vi "PH_PP_CurrentMeas_RT_Startup.vi"() -> ()   [LabVIEW 2014]
uses:
  <vilib>/Utility/error.llb/DialogType.ctl
  <vilib>/DAQmx/create/channels.llb/DAQmx Create Channel (AI-Voltage-Basic).vi
  <vilib>/DAQmx/configure/timing.llb/DAQmx Timing (Sample Clock).vi
  <vilib>/DAQmx/configure/trigger.llb/DAQmx Start Trigger (Analog Edge).vi
  <vilib>/DAQmx/read.llb/DAQmx Read (Analog 1D Wfm NChan NSamp).vi
panel:
  out "Error Port 6343":string
  out "Status Port 6343":string
  out "Error Port 6342":string
  out "Status Port 6342":string
  in  "NI6071E Command Cluster":T1
  in  "error in":errorcluster
  out "Status Port 6341":string
  out "Error Port 6341":string
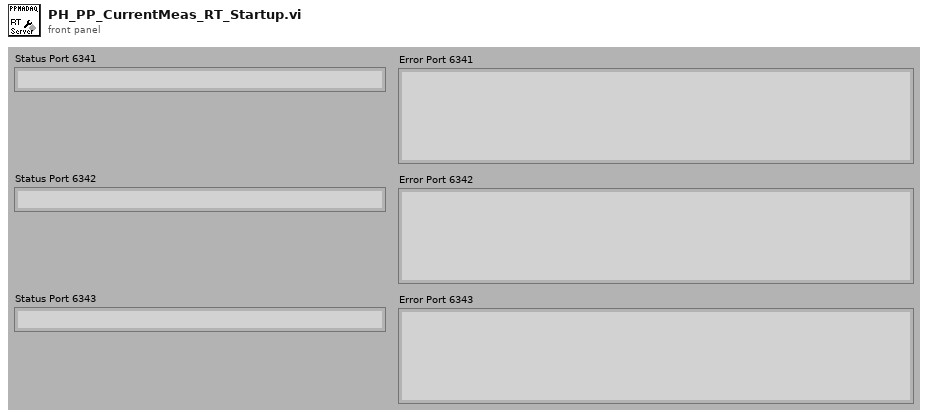
[diagram p1: front panel]
types:
  T1 = cluster{"Command":string, "Data":string, "error out":errorcluster}
  T2 = typedef "DialogType.ctl" = u16
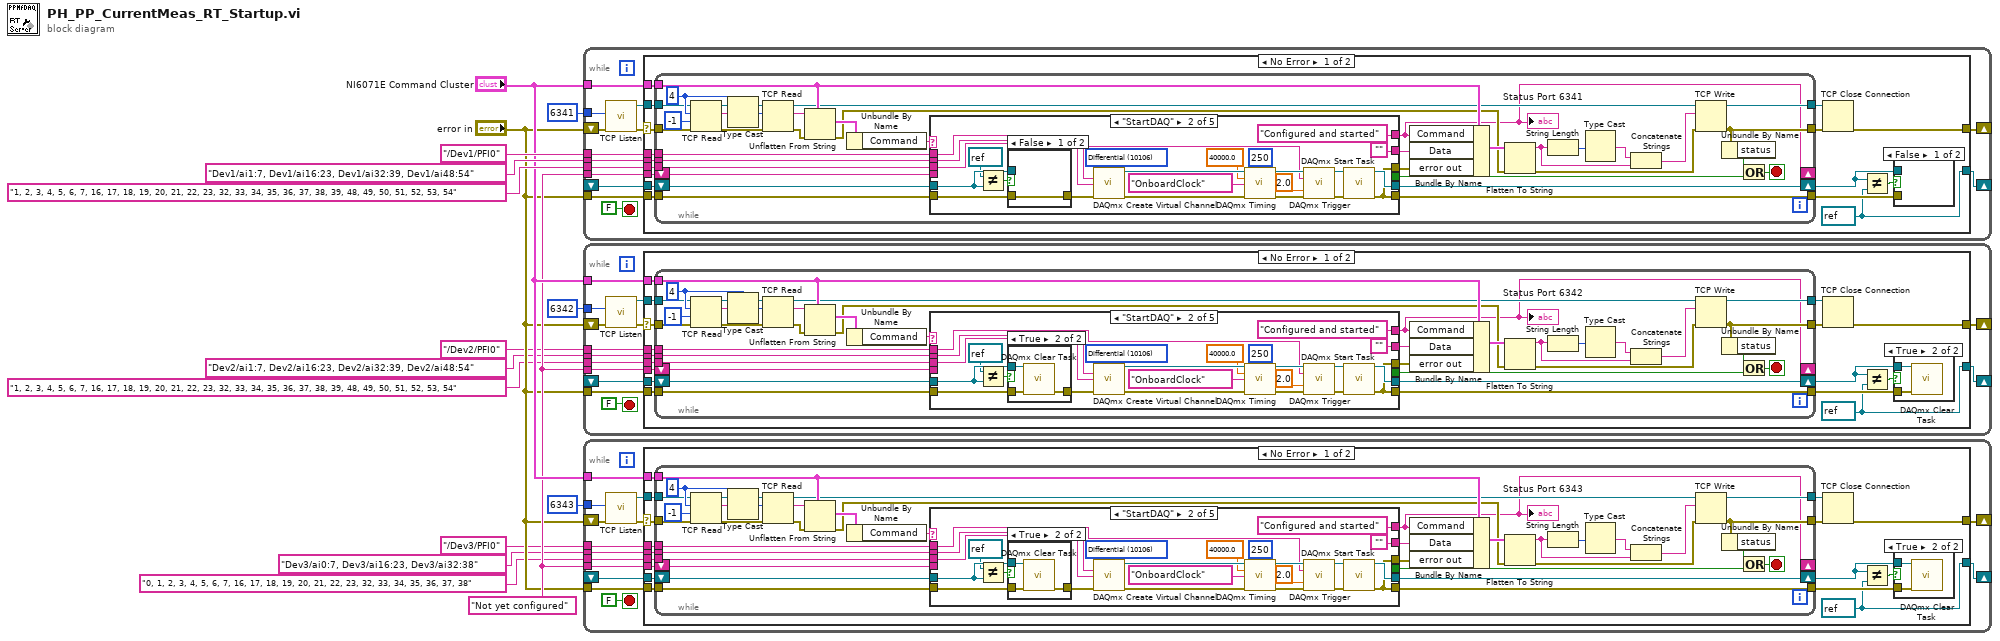
[diagram p0: block diagram]
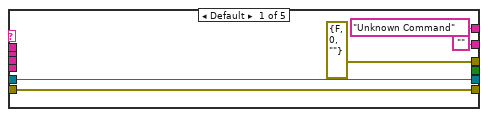
[diagram p3: hidden frame]
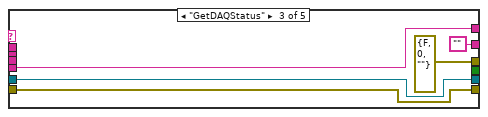
[diagram p5: hidden frame]
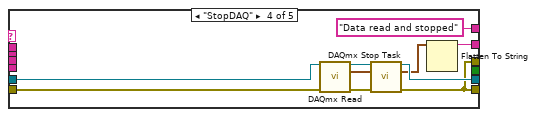
[diagram p6: hidden frame]
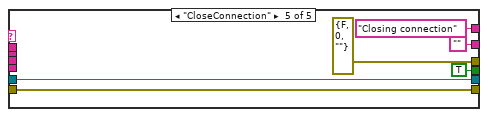
[diagram p7: hidden frame]
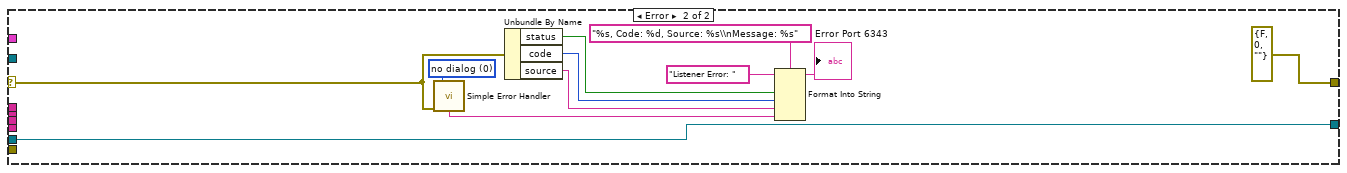
[diagram p8: hidden frame]
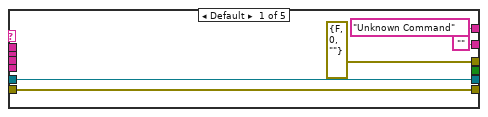
[diagram p10: hidden frame]
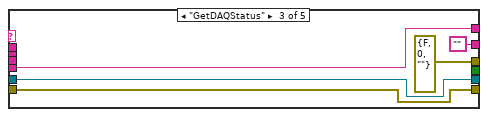
[diagram p12: hidden frame]
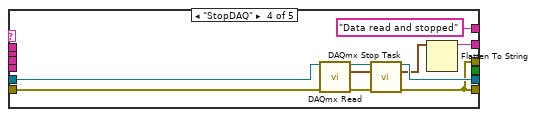
[diagram p13: hidden frame]
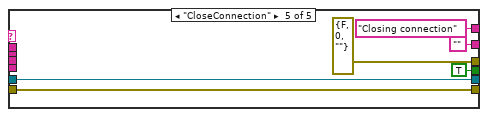
[diagram p14: hidden frame]
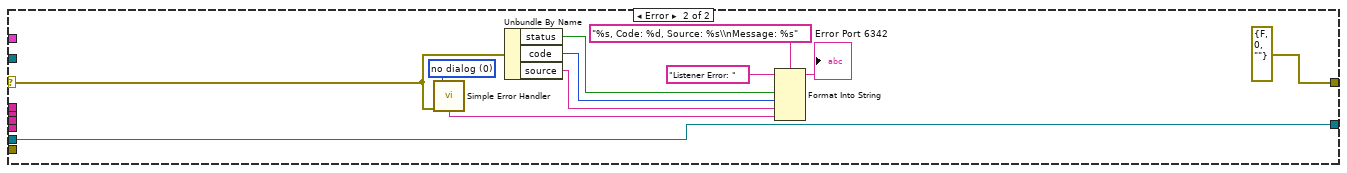
[diagram p15: hidden frame]
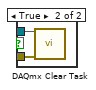
[diagram p16: hidden frame]
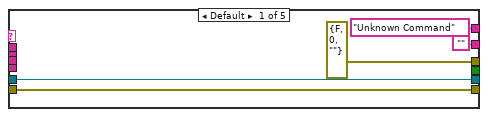
[diagram p17: hidden frame]
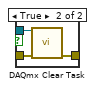
[diagram p18: hidden frame]
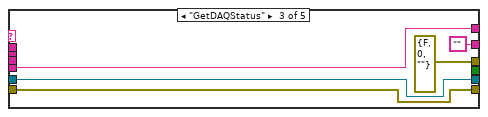
[diagram p19: hidden frame]
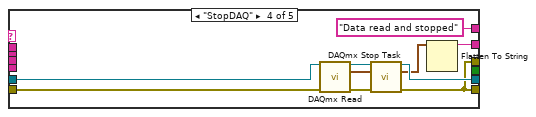
[diagram p20: hidden frame]
diagram:
  w8 = "Not yet configured"
  n1 = while "Main Loop - Wait for Client" {
    tunnel: u16 6341 ("Port") -> [w29]
    shift-right: [w24] -> _
    shift-left: "error in" -> [w25]
    shift-right: [w22] -> _
    shift-left: _ -> [w23]
    tunnel: "error in" -> [w21]
    tunnel: w8 -> [w20]
    tunnel: "NI6071E Command Cluster" -> [w19]
    tunnel: tag "Dev1/ai1:7, Dev1/ai16:23, Dev1/ai32:39, Dev1/ai48:54" ("physical channels (Example given)") -> [w18]
    tunnel: "1, 2, 3, 4, 5, 6, 7, 16, 17, 18, 19, 20, 21, 22, 23, 32, 33, 34, 35, 36, 37, 38, 39, 48, 49, 50, 51, 52, 53, 54" ("name to assign (Example given)") -> [w17]
    tunnel: "/Dev1/PFI0" ("NI6061E Trigger.source (PFI0)") -> [w16]
    stop <- FALSE stop-if-true
    n2 = call <vilib>:"TCP Listen.vi"("error in (no error)"=w25, "port"=w29) -> ("error out"=w28:errorcluster, "connection ID"=w26:refnum<k5>)  [unwired: 5 in, 3 out]
    n3 = case shown="No Error" w28 {
      selector: w28 -> [w44 w140]
      tunnel: w26 -> [w45 _]
      tunnel: [w42 errorcluster {"status"=FALSE, "code"=0, "source"=""} ("error out")] -> w24
      tunnel: w23 -> [w40 w138]
      tunnel: [w34 w138] -> w22
      tunnel: w21 -> [w36 _]
      tunnel: w20 -> [w35 _]
      tunnel: w19 -> [w33 _]
      tunnel: w18 -> [w32 _]
      tunnel: w17 -> [w31 _]
      tunnel: w16 -> [w30 _]
      frame No Error {
        w34 = refnum<k21> refnum ("task in")
        n4 = while "Command Loop" {
          tunnel: w45 -> [w65]
          tunnel: w44 -> [w64]
          tunnel: [w53] -> w43
          tunnel: [w51] -> w41
          tunnel: w36 -> [w81]
          tunnel: [w82] -> w37
          shift-right: [w77] -> w38
          shift-left: w40 -> [w79]
          shift-right: [w48] -> _
          shift-left: w35 -> [w80]
          tunnel: w33 -> [w63]
          tunnel: w32 -> [w74]
          tunnel: w31 -> [w73]
          tunnel: w30 -> [w50]
          stop <- w83 stop-if-true
          w69 = 4 ("bytes to read")
          n5 = TCP Read(connection ID=w65, bytes to read=w69, error in (no error)=w64, 9:-1 ("timeout ms (25000)")) -> (connection ID out=w68:refnum<k5>, data out=w71:string, error out=w67:errorcluster)  [unwired: 1 in]
          n6 = Type Cast(type=w69, x=w71) -> (*(type *) &x=w70:i32)
          n7 = TCP Read(connection ID=w68, bytes to read=w70, error in (no error)=w67) -> (connection ID out=w54:refnum<k5>, data out=w66:string, error out=w61:errorcluster)  [unwired: 2 in]
          n8 = Unflatten From String(type=w63, binary string=w66, error in (no error)=w61) -> (value=w62:T1, error out=w49:errorcluster)  [unwired: 2 in, 1 out]
          n9 = Unbundle By Name(w62) -> ("Command"=w78:string)
          n10 = case shown="\"StartDAQ\"" w78 {
            tunnel: [_ _ _ _ TRUE] -> w84
            tunnel: w79 -> [w85 w94 w117 w125 w135]
            tunnel: [w85 w111 w117 w129 w135] -> w77
            tunnel: [w89 w110 w118 w127 w134] -> w82
            tunnel: w81 -> [w89 w101 w118 w126 w134]
            tunnel: ["Unknown Command" "Configured and started" w119 "Data read and stopped" "Closing connection"] -> w48
            tunnel: w80 -> [_ _ w119 _ _]
            tunnel: [errorcluster {"status"=FALSE, "code"=0, "source"=""} ("error out") w110 errorcluster {"status"=FALSE, "code"=0, "source"=""} ("error out") w127 errorcluster {"status"=FALSE, "code"=0, "source"=""} ("error out")] -> w76
            tunnel: ["" ("data string") "" ("data string") "" ("data string") w128 "" ("data string")] -> w75
            tunnel: w74 -> [_ w91 _ _ _]
            tunnel: w73 -> [_ w90 _ _ _]
            tunnel: w50 -> [_ w92 _ _ _]
            frame Default {
            }
            frame "StartDAQ" {
              w100 = 10106 items=["default"=-1, "RSE"=10083, "NRSE"=10078, "Differential"=10106, "Pseudodifferential"=12529] ("input terminal configuration")
              n11 = Not Equal?(x=refnum<k21> refnum ("y"), y=w94) -> (x != y?=w109:bool)
              n12 = case shown="False" w109 {
                tunnel: w94 -> [_ w115]
                tunnel: w101 -> [w113 w116]
                tunnel: [w113 w114] -> w106
                frame False {
                }
                frame True {
                  n13 = call <vilib>:"DAQmx Clear Task.vi"("task in"=w115, "error in"=w116) -> ("error out"=w114:errorcluster)  [unwired: 13 in]
                }
              }
              n14 = call-poly <vilib>:"DAQmx Create Virtual Channel.vi"("input terminal configuration"=w100, "physical channels"=w91, "name to assign"=w90, "error in"=w106) -> ("task out"=w105:refnum<k21>, "error out"=w104:errorcluster)  [unwired: 10 in]
              n15 = call-poly <vilib>:"DAQmx Timing.vi"("task/channels in"=w105, "samples per channel"=250, "rate"=40000.0, "source"=tag "OnboardClock", "error in"=w104) -> ("task out"=w108:refnum<k21>, "error out"=w107:errorcluster)  [unwired: 9 in]
              n16 = call-poly <vilib>:"DAQmx Trigger.vi"("task/channels in"=w108, "source"=w92, "level"=2.0, "error in"=w107) -> ("task out"=w103:refnum<k21>, "error out"=w102:errorcluster)  [unwired: 10 in]
              n17 = call <vilib>:"DAQmx Start Task.vi"("task/channels in"=w103, "error in"=w102) -> ("task out"=w111:refnum<k21>, "error out"=w110:errorcluster)  [unwired: 12 in]
            }
            frame "GetDAQStatus" {
            }
            frame "StopDAQ" {
              n18 = call-poly <vilib>:"DAQmx Read.vi"("task/channels in"=w125, "error in"=w126) -> ("task out"=w123:refnum<k21>, "data"=w122:waveform(dbl)[], "error out"=w124:errorcluster)  [unwired: 11 in]
              n19 = call <vilib>:"DAQmx Stop Task.vi"("task/channels in"=w123, "error in"=w124) -> ("task out"=w129:refnum<k21>, "error out"=w127:errorcluster)  [unwired: 12 in]
              n20 = Flatten To String(anything=w122) -> (data string=w128:string)  [unwired: 3 in, 2 out]
            }
            frame "CloseConnection" {
            }
          }
          "Status Port 6341" <- w48
          n21 = Bundle By Name(cluster=w63, "Command"=w48, "Data"=w75, "error out"=w76) -> (w55:T1)
          n22 = Flatten To String(anything=w55, error in (no error)=w49) -> (data string=w60:string, error out=w56:errorcluster)  [unwired: 2 in, 1 out]
          n23 = String Length(string=w60) -> (length=w57:i32)
          n24 = Type Cast(x=w57) -> (*(type *) &x=w58:string)  [unwired: 1 in]
          n25 = Concatenate Strings(w58, w60) -> (w59:string)
          n26 = TCP Write(connection ID=w54, data in=w59, error in (no error)=w56) -> (connection ID out=w53:refnum<k5>, error out=w51:errorcluster)  [unwired: 1 in, 1 out]
          n27 = Unbundle By Name(w51) -> ("status"=w52:bool)
          n28 = Or(x=w52, y=w84) -> (x .or. y?=w83:bool)
        }
        n29 = TCP Close Connection(connection ID=w43, error in (no error)=w41) -> (error out=w42:errorcluster)  [unwired: 1 in, 1 out]
        n30 = Not Equal?(x=w38, y=w34) -> (x != y?=w39:bool)
        n31 = case shown="False" w39 {
          tunnel: w38 -> [_ w46]
          tunnel: w37 -> [_ w47]
          frame False {
          }
          frame True {
            n32 = call <vilib>:"DAQmx Clear Task.vi"("task in"=w46, "error in"=w47) -> ()  [unwired: 13 in, 1 out]
          }
        }
      }
      frame Error {
        w142 = T2 0 items=["no dialog", "OK message", "continue or stop message", "OK message + warnings", "continue/stop + warnings"] ("type of dialog (OK msg:1)")
        n33 = call <vilib>:"Simple Error Handler.vi"("type of dialog (OK msg:1)"=w142, "error in (no error)"=w140) -> ("message"=w141:string)  [unwired: 3 in, 4 out]
        n34 = Unbundle By Name(w140) -> ("status"=w147:bool, "code"=w146:i32, "source"=w145:string)
        n35 = Format Into String(format string="%s, Code: %d, Source: %s\\nMessage: %s", initial string="Listener Error: ", w147, w146, w145, w141) -> (resulting string=→"Error Port 6341":string)  [unwired: 1 in, 1 out]
      }
    }
  }
  n36 = while "Main Loop - Wait for Client" {
    tunnel: u16 6342 ("Port") -> [w161]
    shift-right: [w156] -> _
    shift-left: "error in" -> [w157]
    shift-right: [w154] -> _
    shift-left: _ -> [w155]
    tunnel: "error in" -> [w153]
    tunnel: w8 -> [w152]
    tunnel: "NI6071E Command Cluster" -> [w151]
    tunnel: tag "Dev2/ai1:7, Dev2/ai16:23, Dev2/ai32:39, Dev2/ai48:54" ("physical channels (Example given)") -> [w150]
    tunnel: "1, 2, 3, 4, 5, 6, 7, 16, 17, 18, 19, 20, 21, 22, 23, 32, 33, 34, 35, 36, 37, 38, 39, 48, 49, 50, 51, 52, 53, 54" ("name to assign (Example given)") -> [w149]
    tunnel: "/Dev2/PFI0" ("NI6061E Trigger.source (PFI0)") -> [w148]
    stop <- FALSE stop-if-true
    n37 = call <vilib>:"TCP Listen.vi"("error in (no error)"=w157, "port"=w161) -> ("error out"=w160:errorcluster, "connection ID"=w158:refnum<k5>)  [unwired: 5 in, 3 out]
    n38 = case shown="No Error" w160 {
      selector: w160 -> [w176 w272]
      tunnel: w158 -> [w177 _]
      tunnel: [w174 errorcluster {"status"=FALSE, "code"=0, "source"=""} ("error out")] -> w156
      tunnel: w155 -> [w172 w270]
      tunnel: [w166 w270] -> w154
      tunnel: w153 -> [w168 _]
      tunnel: w152 -> [w167 _]
      tunnel: w151 -> [w165 _]
      tunnel: w150 -> [w164 _]
      tunnel: w149 -> [w163 _]
      tunnel: w148 -> [w162 _]
      frame No Error {
        w166 = refnum<k21> refnum ("task in")
        n39 = while "Command Loop" {
          tunnel: w177 -> [w197]
          tunnel: w176 -> [w196]
          tunnel: [w185] -> w175
          tunnel: [w183] -> w173
          tunnel: w168 -> [w213]
          tunnel: [w214] -> w169
          shift-right: [w209] -> w170
          shift-left: w172 -> [w211]
          shift-right: [w180] -> _
          shift-left: w167 -> [w212]
          tunnel: w165 -> [w195]
          tunnel: w164 -> [w206]
          tunnel: w163 -> [w205]
          tunnel: w162 -> [w182]
          stop <- w215 stop-if-true
          w201 = 4 ("bytes to read")
          n40 = TCP Read(connection ID=w197, bytes to read=w201, error in (no error)=w196, 9:-1 ("timeout ms (25000)")) -> (connection ID out=w200:refnum<k5>, data out=w203:string, error out=w199:errorcluster)  [unwired: 1 in]
          n41 = Type Cast(type=w201, x=w203) -> (*(type *) &x=w202:i32)
          n42 = TCP Read(connection ID=w200, bytes to read=w202, error in (no error)=w199) -> (connection ID out=w186:refnum<k5>, data out=w198:string, error out=w193:errorcluster)  [unwired: 2 in]
          n43 = Unflatten From String(type=w195, binary string=w198, error in (no error)=w193) -> (value=w194:T1, error out=w181:errorcluster)  [unwired: 2 in, 1 out]
          n44 = Unbundle By Name(w194) -> ("Command"=w210:string)
          n45 = case shown="\"StartDAQ\"" w210 {
            tunnel: [_ _ _ _ TRUE] -> w216
            tunnel: w211 -> [w217 w226 w249 w257 w267]
            tunnel: [w217 w243 w249 w261 w267] -> w209
            tunnel: [w221 w242 w250 w259 w266] -> w214
            tunnel: w213 -> [w221 w233 w250 w258 w266]
            tunnel: ["Unknown Command" "Configured and started" w251 "Data read and stopped" "Closing connection"] -> w180
            tunnel: w212 -> [_ _ w251 _ _]
            tunnel: [errorcluster {"status"=FALSE, "code"=0, "source"=""} ("error out") w242 errorcluster {"status"=FALSE, "code"=0, "source"=""} ("error out") w259 errorcluster {"status"=FALSE, "code"=0, "source"=""} ("error out")] -> w208
            tunnel: ["" ("data string") "" ("data string") "" ("data string") w260 "" ("data string")] -> w207
            tunnel: w206 -> [_ w223 _ _ _]
            tunnel: w205 -> [_ w222 _ _ _]
            tunnel: w182 -> [_ w224 _ _ _]
            frame Default {
            }
            frame "StartDAQ" {
              w232 = 10106 items=["default"=-1, "RSE"=10083, "NRSE"=10078, "Differential"=10106, "Pseudodifferential"=12529] ("input terminal configuration")
              n46 = Not Equal?(x=refnum<k21> refnum ("y"), y=w226) -> (x != y?=w241:bool)
              n47 = case shown="True" w241 {
                tunnel: w226 -> [_ w247]
                tunnel: w233 -> [w245 w248]
                tunnel: [w245 w246] -> w238
                frame False {
                }
                frame True {
                  n48 = call <vilib>:"DAQmx Clear Task.vi"("task in"=w247, "error in"=w248) -> ("error out"=w246:errorcluster)  [unwired: 13 in]
                }
              }
              n49 = call-poly <vilib>:"DAQmx Create Virtual Channel.vi"("input terminal configuration"=w232, "physical channels"=w223, "name to assign"=w222, "error in"=w238) -> ("task out"=w237:refnum<k21>, "error out"=w236:errorcluster)  [unwired: 10 in]
              n50 = call-poly <vilib>:"DAQmx Timing.vi"("task/channels in"=w237, "samples per channel"=250, "rate"=40000.0, "source"=tag "OnboardClock", "error in"=w236) -> ("task out"=w240:refnum<k21>, "error out"=w239:errorcluster)  [unwired: 9 in]
              n51 = call-poly <vilib>:"DAQmx Trigger.vi"("task/channels in"=w240, "source"=w224, "level"=2.0, "error in"=w239) -> ("task out"=w235:refnum<k21>, "error out"=w234:errorcluster)  [unwired: 10 in]
              n52 = call <vilib>:"DAQmx Start Task.vi"("task/channels in"=w235, "error in"=w234) -> ("task out"=w243:refnum<k21>, "error out"=w242:errorcluster)  [unwired: 12 in]
            }
            frame "GetDAQStatus" {
            }
            frame "StopDAQ" {
              n53 = call-poly <vilib>:"DAQmx Read.vi"("task/channels in"=w257, "error in"=w258) -> ("task out"=w255:refnum<k21>, "data"=w254:waveform(dbl)[], "error out"=w256:errorcluster)  [unwired: 11 in]
              n54 = call <vilib>:"DAQmx Stop Task.vi"("task/channels in"=w255, "error in"=w256) -> ("task out"=w261:refnum<k21>, "error out"=w259:errorcluster)  [unwired: 12 in]
              n55 = Flatten To String(anything=w254) -> (data string=w260:string)  [unwired: 3 in, 2 out]
            }
            frame "CloseConnection" {
            }
          }
          "Status Port 6342" <- w180
          n56 = Bundle By Name(cluster=w195, "Command"=w180, "Data"=w207, "error out"=w208) -> (w187:T1)
          n57 = Flatten To String(anything=w187, error in (no error)=w181) -> (data string=w192:string, error out=w188:errorcluster)  [unwired: 2 in, 1 out]
          n58 = String Length(string=w192) -> (length=w189:i32)
          n59 = Type Cast(x=w189) -> (*(type *) &x=w190:string)  [unwired: 1 in]
          n60 = Concatenate Strings(w190, w192) -> (w191:string)
          n61 = TCP Write(connection ID=w186, data in=w191, error in (no error)=w188) -> (connection ID out=w185:refnum<k5>, error out=w183:errorcluster)  [unwired: 1 in, 1 out]
          n62 = Unbundle By Name(w183) -> ("status"=w184:bool)
          n63 = Or(x=w184, y=w216) -> (x .or. y?=w215:bool)
        }
        n64 = TCP Close Connection(connection ID=w175, error in (no error)=w173) -> (error out=w174:errorcluster)  [unwired: 1 in, 1 out]
        n65 = Not Equal?(x=w170, y=w166) -> (x != y?=w171:bool)
        n66 = case shown="True" w171 {
          tunnel: w170 -> [_ w178]
          tunnel: w169 -> [_ w179]
          frame False {
          }
          frame True {
            n67 = call <vilib>:"DAQmx Clear Task.vi"("task in"=w178, "error in"=w179) -> ()  [unwired: 13 in, 1 out]
          }
        }
      }
      frame Error {
        w274 = T2 0 items=["no dialog", "OK message", "continue or stop message", "OK message + warnings", "continue/stop + warnings"] ("type of dialog (OK msg:1)")
        n68 = call <vilib>:"Simple Error Handler.vi"("type of dialog (OK msg:1)"=w274, "error in (no error)"=w272) -> ("message"=w273:string)  [unwired: 3 in, 4 out]
        n69 = Unbundle By Name(w272) -> ("status"=w279:bool, "code"=w278:i32, "source"=w277:string)
        n70 = Format Into String(format string="%s, Code: %d, Source: %s\\nMessage: %s", initial string="Listener Error: ", w279, w278, w277, w273) -> (resulting string=→"Error Port 6342":string)  [unwired: 1 in, 1 out]
      }
    }
  }
  n71 = while "Main Loop - Wait for Client" {
    tunnel: u16 6343 ("Port") -> [w293]
    shift-right: [w288] -> _
    shift-left: "error in" -> [w289]
    shift-right: [w286] -> _
    shift-left: _ -> [w287]
    tunnel: "error in" -> [w285]
    tunnel: w8 -> [w284]
    tunnel: "NI6071E Command Cluster" -> [w283]
    tunnel: tag "Dev3/ai0:7, Dev3/ai16:23, Dev3/ai32:38" ("physical channels (Example given)") -> [w282]
    tunnel: "0, 1, 2, 3, 4, 5, 6, 7, 16, 17, 18, 19, 20, 21, 22, 23, 32, 33, 34, 35, 36, 37, 38" ("name to assign (Example given)") -> [w281]
    tunnel: "/Dev3/PFI0" ("NI6061E Trigger.source (PFI0)") -> [w280]
    stop <- FALSE stop-if-true
    n72 = call <vilib>:"TCP Listen.vi"("error in (no error)"=w289, "port"=w293) -> ("error out"=w292:errorcluster, "connection ID"=w290:refnum<k5>)  [unwired: 5 in, 3 out]
    n73 = case shown="No Error" w292 {
      selector: w292 -> [w308 w404]
      tunnel: w290 -> [w309 _]
      tunnel: [w306 errorcluster {"status"=FALSE, "code"=0, "source"=""} ("error out")] -> w288
      tunnel: w287 -> [w304 w402]
      tunnel: [w298 w402] -> w286
      tunnel: w285 -> [w300 _]
      tunnel: w284 -> [w299 _]
      tunnel: w283 -> [w297 _]
      tunnel: w282 -> [w296 _]
      tunnel: w281 -> [w295 _]
      tunnel: w280 -> [w294 _]
      frame No Error {
        w298 = refnum<k21> refnum ("task in")
        n74 = while "Command Loop" {
          tunnel: w309 -> [w329]
          tunnel: w308 -> [w328]
          tunnel: [w317] -> w307
          tunnel: [w315] -> w305
          tunnel: w300 -> [w345]
          tunnel: [w346] -> w301
          shift-right: [w341] -> w302
          shift-left: w304 -> [w343]
          shift-right: [w312] -> _
          shift-left: w299 -> [w344]
          tunnel: w297 -> [w327]
          tunnel: w296 -> [w338]
          tunnel: w295 -> [w337]
          tunnel: w294 -> [w314]
          stop <- w347 stop-if-true
          w333 = 4 ("bytes to read")
          n75 = TCP Read(connection ID=w329, bytes to read=w333, error in (no error)=w328, 9:-1 ("timeout ms (25000)")) -> (connection ID out=w332:refnum<k5>, data out=w335:string, error out=w331:errorcluster)  [unwired: 1 in]
          n76 = Type Cast(type=w333, x=w335) -> (*(type *) &x=w334:i32)
          n77 = TCP Read(connection ID=w332, bytes to read=w334, error in (no error)=w331) -> (connection ID out=w318:refnum<k5>, data out=w330:string, error out=w325:errorcluster)  [unwired: 2 in]
          n78 = Unflatten From String(type=w327, binary string=w330, error in (no error)=w325) -> (value=w326:T1, error out=w313:errorcluster)  [unwired: 2 in, 1 out]
          n79 = Unbundle By Name(w326) -> ("Command"=w342:string)
          n80 = case shown="\"StartDAQ\"" w342 {
            tunnel: [_ _ _ _ TRUE] -> w348
            tunnel: w343 -> [w349 w358 w381 w389 w399]
            tunnel: [w349 w375 w381 w393 w399] -> w341
            tunnel: [w353 w374 w382 w391 w398] -> w346
            tunnel: w345 -> [w353 w365 w382 w390 w398]
            tunnel: ["Unknown Command" "Configured and started" w383 "Data read and stopped" "Closing connection"] -> w312
            tunnel: w344 -> [_ _ w383 _ _]
            tunnel: [errorcluster {"status"=FALSE, "code"=0, "source"=""} ("error out") w374 errorcluster {"status"=FALSE, "code"=0, "source"=""} ("error out") w391 errorcluster {"status"=FALSE, "code"=0, "source"=""} ("error out")] -> w340
            tunnel: ["" ("data string") "" ("data string") "" ("data string") w392 "" ("data string")] -> w339
            tunnel: w338 -> [_ w355 _ _ _]
            tunnel: w337 -> [_ w354 _ _ _]
            tunnel: w314 -> [_ w356 _ _ _]
            frame Default {
            }
            frame "StartDAQ" {
              w364 = 10106 items=["default"=-1, "RSE"=10083, "NRSE"=10078, "Differential"=10106, "Pseudodifferential"=12529] ("input terminal configuration")
              n81 = Not Equal?(x=refnum<k21> refnum ("y"), y=w358) -> (x != y?=w373:bool)
              n82 = case shown="True" w373 {
                tunnel: w358 -> [_ w379]
                tunnel: w365 -> [w377 w380]
                tunnel: [w377 w378] -> w370
                frame False {
                }
                frame True {
                  n83 = call <vilib>:"DAQmx Clear Task.vi"("task in"=w379, "error in"=w380) -> ("error out"=w378:errorcluster)  [unwired: 13 in]
                }
              }
              n84 = call-poly <vilib>:"DAQmx Create Virtual Channel.vi"("input terminal configuration"=w364, "physical channels"=w355, "name to assign"=w354, "error in"=w370) -> ("task out"=w369:refnum<k21>, "error out"=w368:errorcluster)  [unwired: 10 in]
              n85 = call-poly <vilib>:"DAQmx Timing.vi"("task/channels in"=w369, "samples per channel"=250, "rate"=40000.0, "source"=tag "OnboardClock", "error in"=w368) -> ("task out"=w372:refnum<k21>, "error out"=w371:errorcluster)  [unwired: 9 in]
              n86 = call-poly <vilib>:"DAQmx Trigger.vi"("task/channels in"=w372, "source"=w356, "level"=2.0, "error in"=w371) -> ("task out"=w367:refnum<k21>, "error out"=w366:errorcluster)  [unwired: 10 in]
              n87 = call <vilib>:"DAQmx Start Task.vi"("task/channels in"=w367, "error in"=w366) -> ("task out"=w375:refnum<k21>, "error out"=w374:errorcluster)  [unwired: 12 in]
            }
            frame "GetDAQStatus" {
            }
            frame "StopDAQ" {
              n88 = call-poly <vilib>:"DAQmx Read.vi"("task/channels in"=w389, "error in"=w390) -> ("task out"=w387:refnum<k21>, "data"=w386:waveform(dbl)[], "error out"=w388:errorcluster)  [unwired: 11 in]
              n89 = call <vilib>:"DAQmx Stop Task.vi"("task/channels in"=w387, "error in"=w388) -> ("task out"=w393:refnum<k21>, "error out"=w391:errorcluster)  [unwired: 12 in]
              n90 = Flatten To String(anything=w386) -> (data string=w392:string)  [unwired: 3 in, 2 out]
            }
            frame "CloseConnection" {
            }
          }
          "Status Port 6343" <- w312
          n91 = Bundle By Name(cluster=w327, "Command"=w312, "Data"=w339, "error out"=w340) -> (w319:T1)
          n92 = Flatten To String(anything=w319, error in (no error)=w313) -> (data string=w324:string, error out=w320:errorcluster)  [unwired: 2 in, 1 out]
          n93 = String Length(string=w324) -> (length=w321:i32)
          n94 = Type Cast(x=w321) -> (*(type *) &x=w322:string)  [unwired: 1 in]
          n95 = Concatenate Strings(w322, w324) -> (w323:string)
          n96 = TCP Write(connection ID=w318, data in=w323, error in (no error)=w320) -> (connection ID out=w317:refnum<k5>, error out=w315:errorcluster)  [unwired: 1 in, 1 out]
          n97 = Unbundle By Name(w315) -> ("status"=w316:bool)
          n98 = Or(x=w316, y=w348) -> (x .or. y?=w347:bool)
        }
        n99 = TCP Close Connection(connection ID=w307, error in (no error)=w305) -> (error out=w306:errorcluster)  [unwired: 1 in, 1 out]
        n100 = Not Equal?(x=w302, y=w298) -> (x != y?=w303:bool)
        n101 = case shown="True" w303 {
          tunnel: w302 -> [_ w310]
          tunnel: w301 -> [_ w311]
          frame False {
          }
          frame True {
            n102 = call <vilib>:"DAQmx Clear Task.vi"("task in"=w310, "error in"=w311) -> ()  [unwired: 13 in, 1 out]
          }
        }
      }
      frame Error {
        w406 = T2 0 items=["no dialog", "OK message", "continue or stop message", "OK message + warnings", "continue/stop + warnings"] ("type of dialog (OK msg:1)")
        n103 = call <vilib>:"Simple Error Handler.vi"("type of dialog (OK msg:1)"=w406, "error in (no error)"=w404) -> ("message"=w405:string)  [unwired: 3 in, 4 out]
        n104 = Unbundle By Name(w404) -> ("status"=w411:bool, "code"=w410:i32, "source"=w409:string)
        n105 = Format Into String(format string="%s, Code: %d, Source: %s\\nMessage: %s", initial string="Listener Error: ", w411, w410, w409, w405) -> (resulting string=→"Error Port 6343":string)  [unwired: 1 in, 1 out]
      }
    }
  }
